vi "Projectile.vi"() -> ()   [LabVIEW 2015]
panel:
  out "R":dbl[](array[numeric])
  out "XY Graph":cluster{dbl[], dbl[]}(graph)
  in  "Launch Height (m)":dbl
  in  "Launch Speed (m/s)":dbl
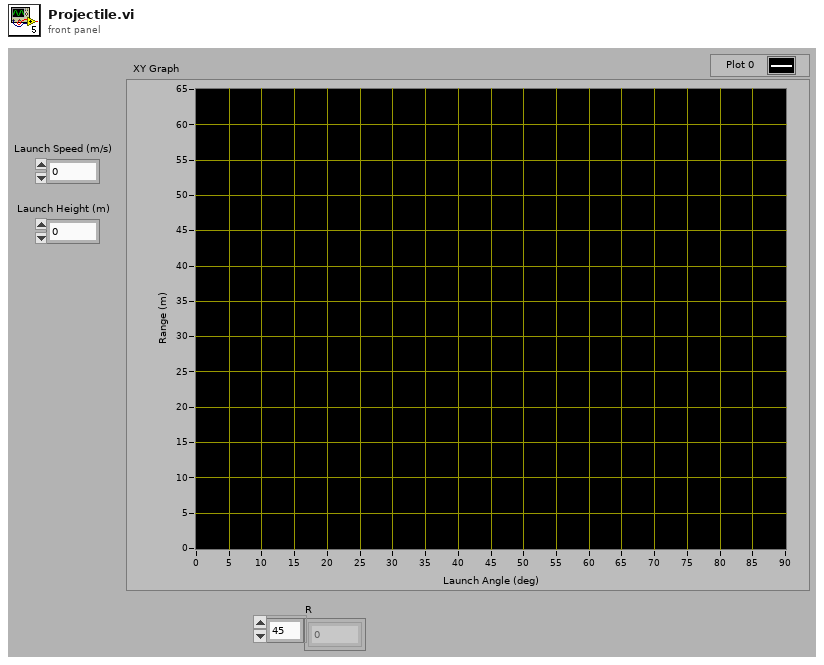
[diagram p1: front panel]
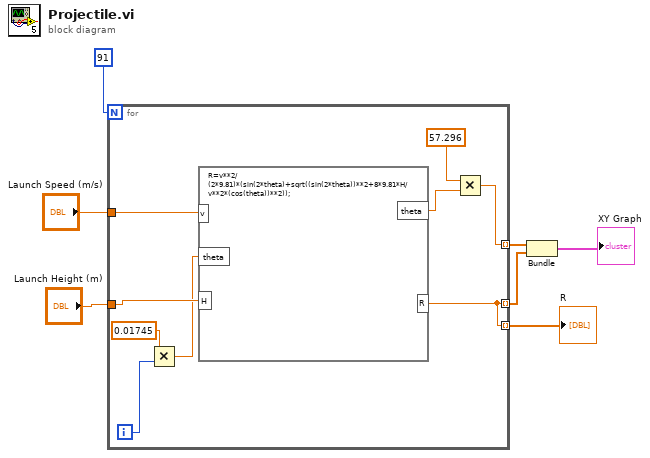
[diagram p0: block diagram]
diagram:
  n1 = for {
    N: 91 -> [_]
    tunnel: "Launch Speed (m/s)" -> [w16]
    tunnel: "Launch Height (m)" -> [w15]
    tunnel: [w8] -> w3 mode=indexing
    tunnel: [w14] -> w2 mode=indexing
    tunnel: [w14] -> w1 mode=indexing
    i -> [w13]
    n2 = Multiply(x=0.01745, y=w13) -> (x*y=w11:dbl)
    n3 = formula code="R=v**2/(2*9.81)*(sin(2*theta)+sqrt((sin(2*theta))**2+8*9.81*H/v**2*(cos(theta))**2));"("v"=w16, "H"=w15, "theta"=w11) -> ("theta"=w9:dbl, "R"=w14:dbl)
    n4 = Multiply(x=57.296, y=w9) -> (x*y=w8:dbl)
  }
  "R" <- w1
  n5 = Bundle(w3, w2) -> (→"XY Graph":cluster{dbl[], dbl[]})  [unwired: 1 in]
